vi "gmail html.vi"(5 "Subject":string="Sending TLS Authenticated Email", 7 "Body":string="<!DOCTYPE html>\n<html>\n<body>\n<!DOCTYPE html>\n<html>\n<body>\n\n<h1>Hi Alex</h1>\n\n<p>Check out the <a href=\"http://aguaclara.cornell.edu\">AguaClara website</a>.</p>\n<p><img src=\"https://lh4.googleusercontent.com/-pjSUYulSdkk/T8OoEFFC3MI/AAAAAAAAnJ4/auIcAqZFd5Q/s1058/IMG_6049.JPG\" alt=\"\" width=\"300\" height=\"200\" /></p> \n<p><a href=\"https://www.giving.cornell.edu/give/?gifttype=1&gifttype2=77&comments=AguaClara%20-%20Account%20E65-8769\">Donate now</a> to make a real difference</p>\n</body> \n</html>\n    \n    \n", 8 "error in (no error)":errorcluster, 9 "Server":T1={"Outgoing Mail Server (SMTP)"="smtp.gmail.com", "MAIL Account User ID"="monroews", "MAIL Account Password"="", "Enable SSL"=TRUE, "Port"=587, "Sender's Email Address"="monroews@gmail.com", "Sender's Name"="Monroe Weber-Shirk"}, 10 "Recipient's Name":string="Monroe", 11 "Recipient's Email Address":string="mw24@cornell.edu") -> (0 "error out":errorcluster)   [LabVIEW 2012]
uses:
  Mail Server.ctl
  ADT 2/AguaClara Library.lvlib
panel:
  in  "IsBodyHtml":bool
  in  "CC (Carbon Copy Recipient - Optional)":string
  in  "Attachment - Optional":path
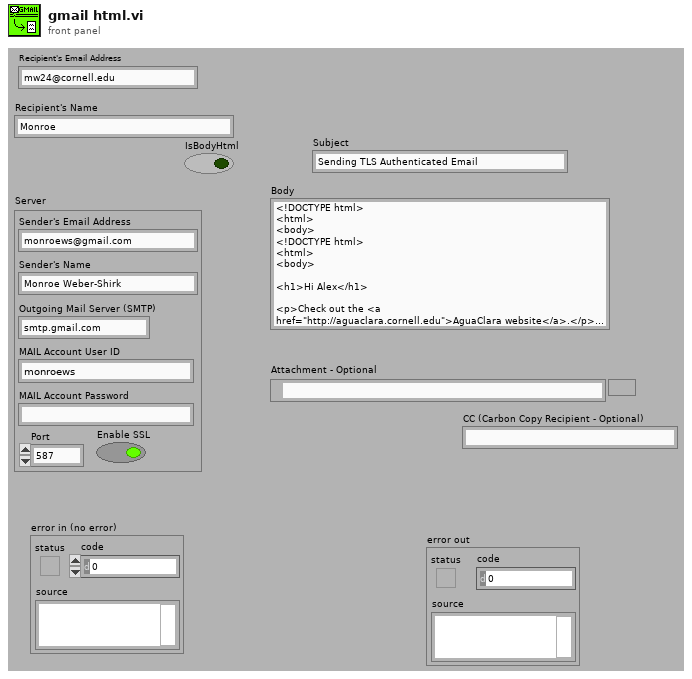
[diagram p1: front panel]
types:
  T1 = typedef "Mail Server.ctl" = cluster{"Outgoing Mail Server (SMTP)":string, "MAIL Account User ID":string, "MAIL Account Password":string, "Enable SSL":bool, "Port":i32, "Sender's Email Address":string, "Sender's Name":string}
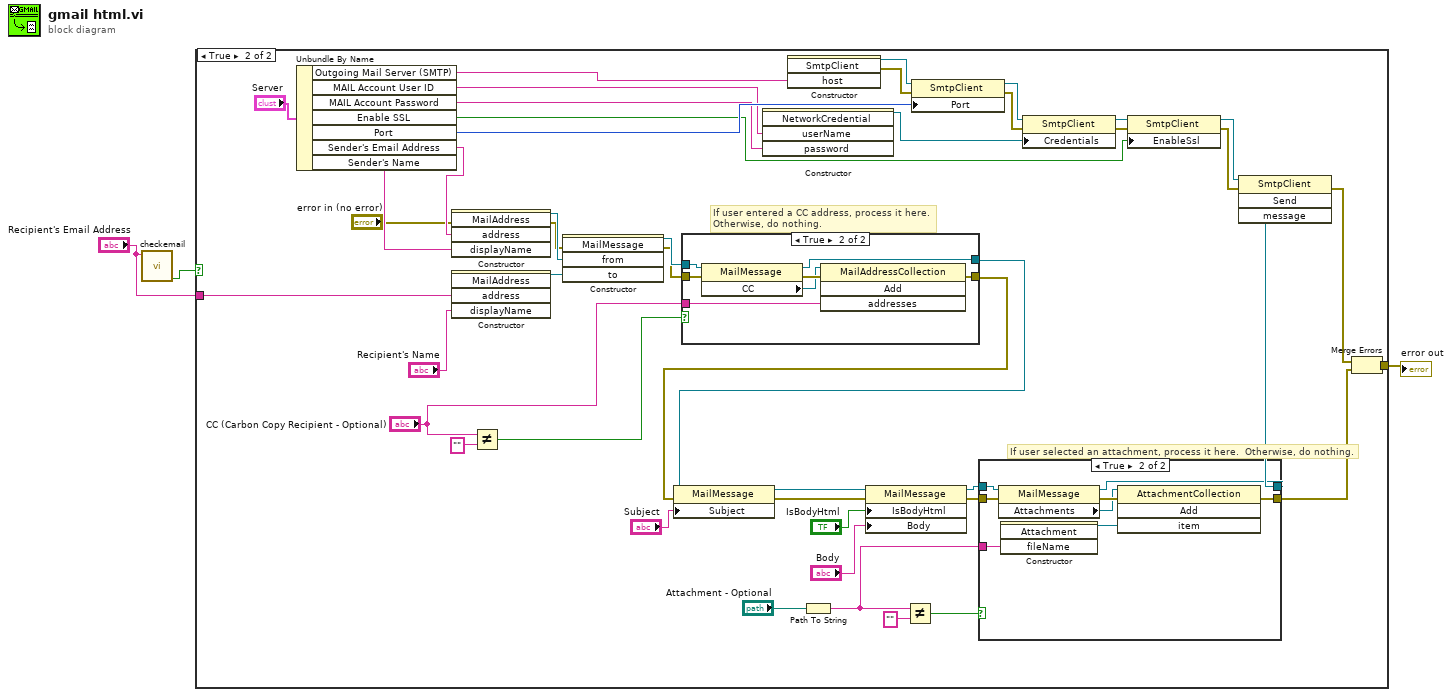
[diagram p0: block diagram]
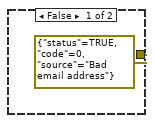
[diagram p2: hidden frame]
diagram:
  n1 = call "checkemail.vi"("email"="Recipient's Email Address") -> ("valid email"=w2:bool)  [unwired: 7 in, 3 out]
  n2 = case shown="True" w2 {
    tunnel: "Recipient's Email Address" -> [_ w11]
    tunnel: [errorcluster {"status"=TRUE, "code"=0, "source"="Bad email address"} ("error IO") w9] -> w1
    frame False {
    }
    frame True {
      # "If user selected an attachment, process it here.  Otherwise, do nothing."
      # "If user entered a CC address, process it here.\nOtherwise, do nothing."
      n3 = Unbundle By Name("Server") -> ("Outgoing Mail Server (SMTP)"=w18:string, "MAIL Account User ID"=w16:string, "MAIL Account Password"=w15:string, "Enable SSL"=w14:bool, "Port"=w17:i32, "Sender's Email Address"=w8:string, "Sender's Name"=w7:string)
      n4 = constructor class="MailAddress"(error in="error in (no error)", "address"=w8, "displayName"=w7) -> (reference out=w48:refnum<k24>, error out=w6:errorcluster)  [unwired: 2 in, 3 out]
      n5 = constructor class="MailAddress"("address"=w11, "displayName"="Recipient's Name") -> (reference out=w49:refnum<k24>)  [unwired: 3 in, 4 out]
      n6 = Not Equal?(x="CC (Carbon Copy Recipient - Optional)", y="") -> (x != y?=w10:bool)
      n7 = constructor class="MailMessage"(error in=w6, "from"=w48, "to"=w49) -> (reference out=w25:refnum<k24>, error out=w24:errorcluster)  [unwired: 2 in, 3 out]
      n8 = case shown="True" w10 {
        tunnel: "CC (Carbon Copy Recipient - Optional)" -> [_ w56]
        tunnel: w25 -> [w51 w55]
        tunnel: w24 -> [w50 w54]
        tunnel: [w51 w53] -> w23
        tunnel: [w50 w52] -> w22
        frame False {
        }
        frame True {
          n9 = property class="MailMessage"(reference=w55, error in=w54) -> (reference out=w53:refnum<k24>, error out=w58:errorcluster, "CC"=w57:refnum<k24>)
          n10 = invoke class="MailAddressCollection" method="Add"(reference=w57, error in=w58, "addresses"=w56) -> (error out=w52:errorcluster)  [unwired: 1 in, 3 out]
        }
      }
      n11 = property class="MailMessage"(reference=w23, error in=w22, "Subject"="Subject") -> (reference out=w43:refnum<k24>, error out=w47:errorcluster)
      n12 = constructor class="NetworkCredential"("userName"=w16, "password"=w15) -> (reference out=w42:refnum<k24>)  [unwired: 3 in, 4 out]
      n13 = constructor class="SmtpClient"("host"=w18) -> (reference out=w41:refnum<k24>, error out=w37:errorcluster)  [unwired: 3 in, 2 out]
      n14 = Path To String(path="Attachment - Optional") -> (string=w28:string)
      n15 = property class="MailMessage"(reference=w43, error in=w47, "IsBodyHtml"="IsBodyHtml", "Body"="Body") -> (reference out=w33:refnum<k24>, error out=w20:errorcluster)
      n16 = Not Equal?(x=w28, y="") -> (x != y?=w29:bool)
      n17 = property class="SmtpClient"(reference=w41, error in=w37, "Port"=w17) -> (reference out=w40:refnum<k24>, error out=w36:errorcluster)
      n18 = case shown="True" w29 {
        tunnel: w33 -> [w60 w65]
        tunnel: [w60 w64] -> w32
        tunnel: w28 -> [_ w63]
        tunnel: w20 -> [w59 w62]
        tunnel: [w59 w61] -> w12
        frame False {
        }
        frame True {
          n19 = property class="MailMessage"(reference=w65, error in=w62) -> (reference out=w64:refnum<k24>, error out=w68:errorcluster, "Attachments"=w66:refnum<k24>)
          n20 = constructor class="Attachment"("fileName"=w63) -> (reference out=w67:refnum<k24>)  [unwired: 3 in, 3 out]
          n21 = invoke class="AttachmentCollection" method="Add"(reference=w66, error in=w68, "item"=w67) -> (error out=w61:errorcluster)  [unwired: 1 in, 3 out]
        }
      }
      n22 = property class="SmtpClient"(reference=w40, error in=w36, "Credentials"=w42) -> (reference out=w39:refnum<k24>, error out=w35:errorcluster)
      n23 = property class="SmtpClient"(reference=w39, error in=w35, "EnableSsl"=w14) -> (reference out=w38:refnum<k24>, error out=w34:errorcluster)
      n24 = invoke class="SmtpClient" method="Send"(reference=w38, error in=w34, "message"=w32) -> (error out=w13:errorcluster)  [unwired: 1 in, 3 out]
      n25 = Merge Errors(w13, w12) -> (w9:errorcluster)
    }
  }
  "error out" <- w1
